vi "Drive Controller.vi"(8 "error in":errorcluster) -> ()   [LabVIEW 2015]
doc: "This VI executes continuously carrying out the current operation and responding to updates or new operation requests. It will often contain the timing or control code that is difficult to place directly in TeleOp. This VI generally opens all sensors and motors and isolates the rest of the robot code from knowing implementation details of how the operations are carried out."
uses:
  Drive Setpoints.ctl
  Drive Operations.ctl
  <vilib>/Rock Robotics/WPI/SafetyOutput/WPI_SafetyOutputConfigMenu.ctl
  <vilib>/Rock Robotics/WPI/RobotDrive/WPI_RobotDriveOpen2MotorWithTalon.vi
panel:
  in  "CMD Limit":dbl=0.07
  out "Setpoints":T1(graph)
  out "Current\nCmd":string
  # "Tip: It may be helpful to observe inputs and sensor values.\nYou may also want to display tuning or debugging controls."
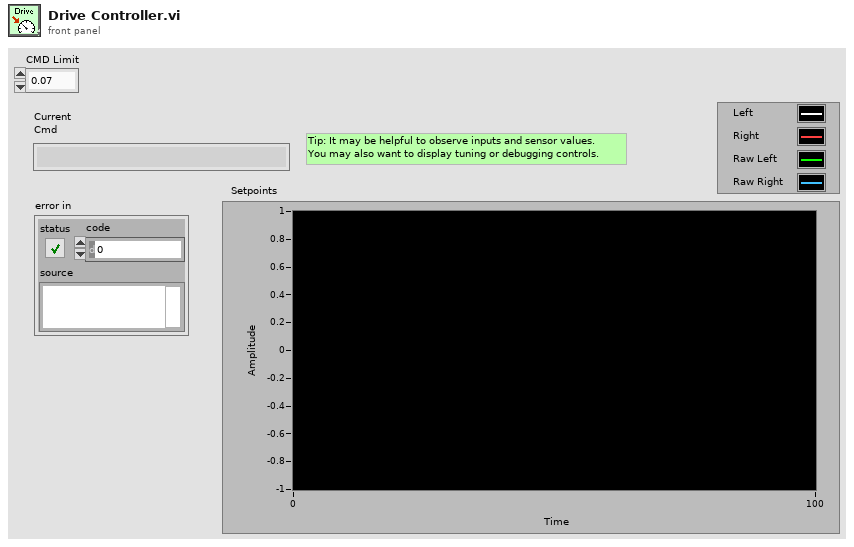
[diagram p1: front panel]
types:
  T1 = cluster{"Don't move motors while reserved":dbl, "Don't move motors while reserved":dbl, "Left Setpoint":dbl, "Right Setpoint":dbl}
  T2 = typedef "WPI_SafetyOutputConfigMenu.ctl" = enum16{"Enable", "Disable"}
  T3 = typedef "Drive Setpoints.ctl" = cluster{"Operation":T4, "Left Setpoint":dbl, "Right Setpoint":dbl, "Duration":dbl, "Throttle Setpoint":dbl}
  T4 = typedef "Drive Operations.ctl" = enum16{"Reserve", "Read Current", "Immediate", "Drive for Time", "Drive for Distance"}
  T5 = typedef "WPI_RobotDriveDevRef.ctl" = cluster{"DevStatus":errorcluster, "Motors[]":T6[], "Square Inputs":bool, "Max Output":dbl}
  T6 = typedef "WPI_MotorControlDeviceRef.ctl" = cluster{"DeviceStatus":errorcluster, "Type":T7, "PWM":cluster{"PWM Channel":T8, "DeadBand":T9}, "CAN":cluster{"Device Number":u8, "Control Mode":T10, "Semaphore":T11, "Max Vout":dbl, "TalonSRX Control Mode":T12}, "Invert":bool}
  T7 = typedef "WPI_MotorControlType.ctl" = enum16{"PWM", "CAN", "CANTalonSRX"}
  T8 = typedef "FPGA_DIOPWMChannel.ctl" = enum8{"PWM 0", "PWM 1", "PWM 2", "PWM 3", "PWM 4", "PWM 5", "PWM 6", "PWM 7", "PWM 8", "PWM 9", "PWM MXP 0", "PWM MXP 1", "PWM MXP 2", "PWM MXP 3", "PWM MXP 4", "PWM MXP 5", "PWM MXP 6", "PWM MXP 7", "PWM MXP 8", "PWM MXP 9", "Invalid"}
  T9 = typedef "WPI_PWMDeadband.ctl" = cluster{"Name":string, "maxPositivePwm":i32, "minPositivePwm":i32, "centerPwm":i32, "maxNegativePwm":i32, "minNegativePwm":i32, "angularRange":u16}
  T10 = typedef "WPI_CANJaguar_ControlMode.ctl" = enum8{"Percent VBus", "Current", "Speed", "Position", "Voltage"}
  T11 = typedef "Semaphore RefNum" = refnum<k1>
  T12 = typedef "WPI_CANTalonSRX_APIControlMode.ctl" = enum8{"Percent VBus", "Speed", "Position", "Slave", "Unchanged / Invalid", "Voltage Compensation", "Current", "Motion Profile"}
  T13 = typedef "Command Status Info.ctl" = cluster{"Name":string, "Status":T14, "notifier out":T15}
  T14 = typedef "Completion Status.ctl" = enum16{"Successful", "Aborted", "Incomplete"}
  T15 = typedef "Completion Notifier.ctl" = refnum<notifier>
  T16 = cluster{"SubSystem Data":T3, cluster{"Start Time (ms)":u32, "Iterations":i32}, cluster{"Command Info":T13, "Description":string, "SubSystem Data":T3, "notifier out":refnum<notifier>, "Subsystem Name":string}}
  T17 = cluster{"SubSystem Data":T3, cluster{"Start Time (ms)":u32, "Iterations":i32}, "Default Command Arguments":cluster{"Command Info":T13, "Description":string, "SubSystem Data":T3, "notifier out":refnum<notifier>, "Subsystem Name":string}}
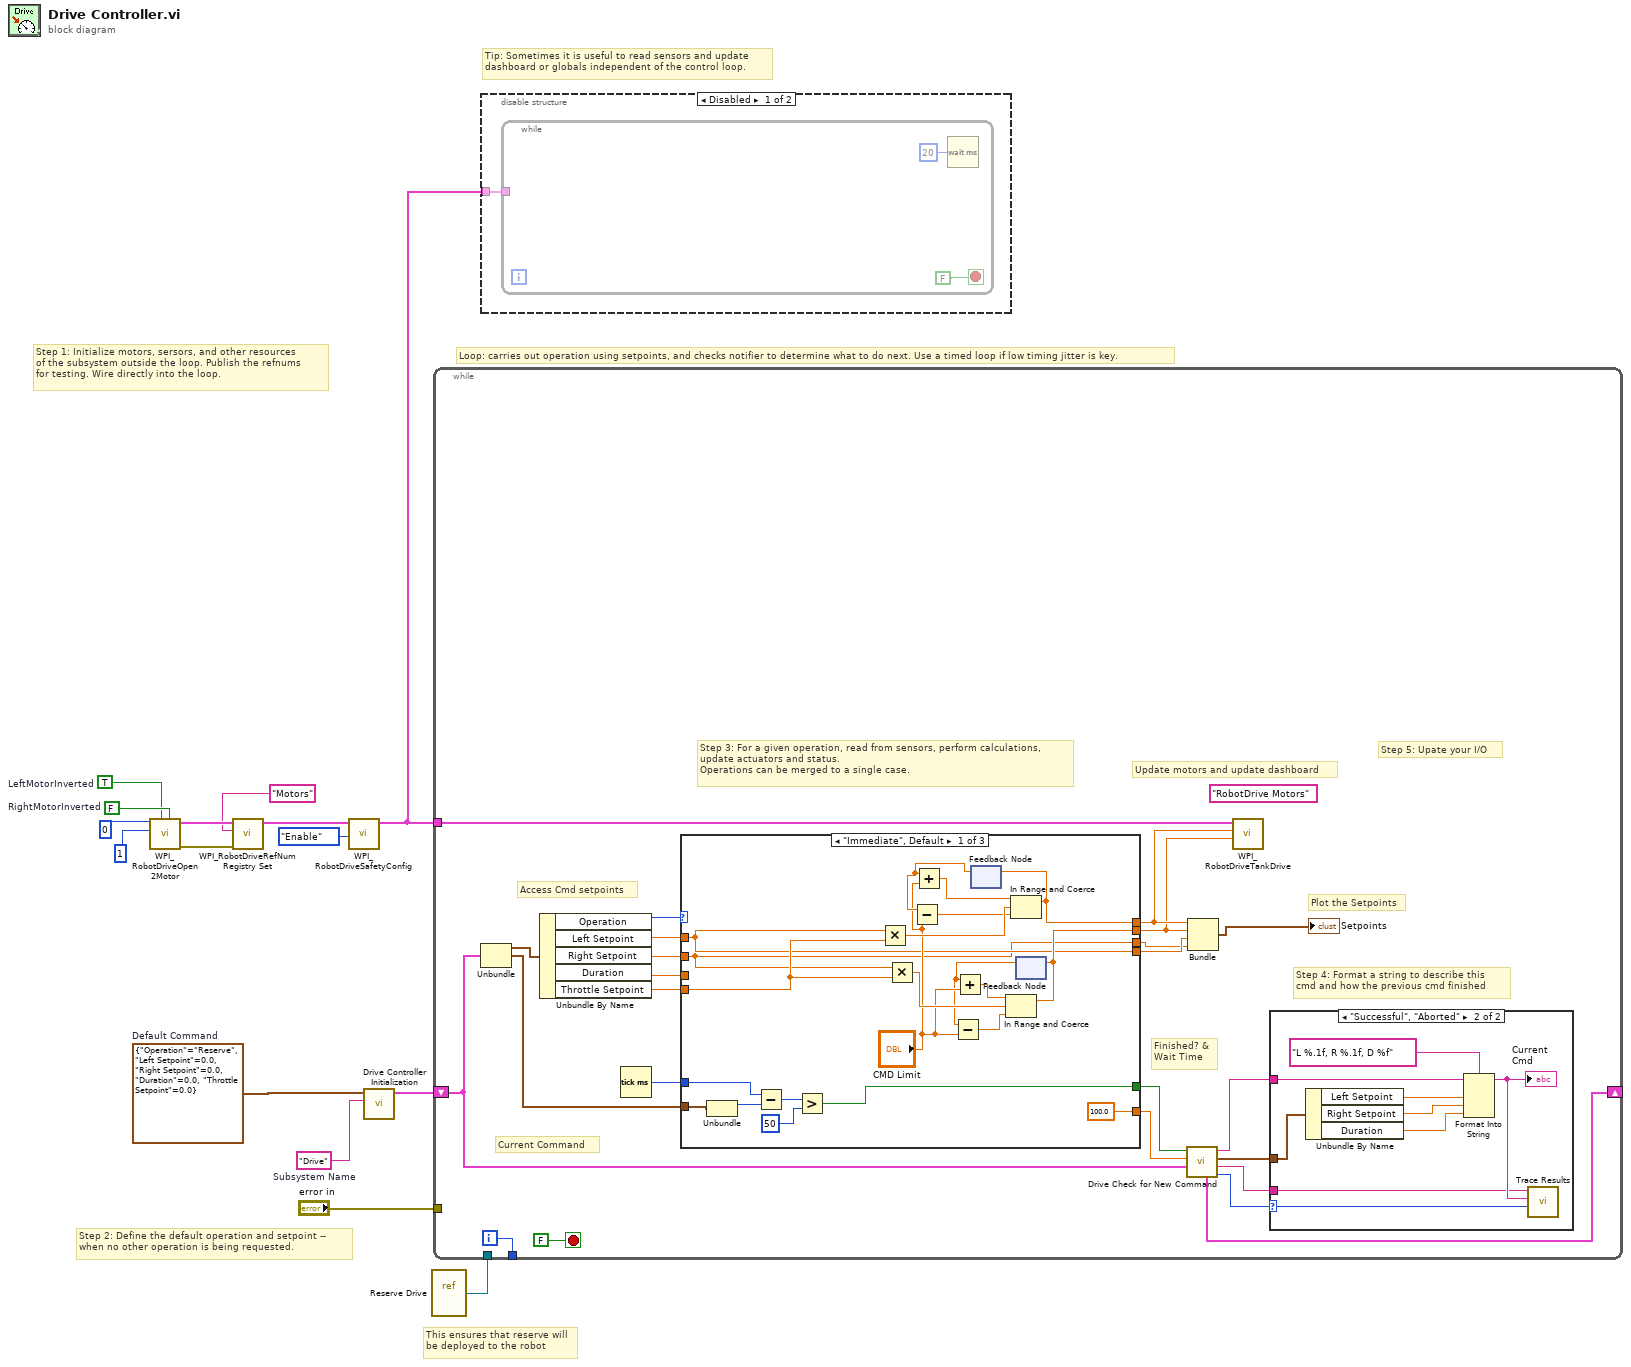
[diagram p0: block diagram]
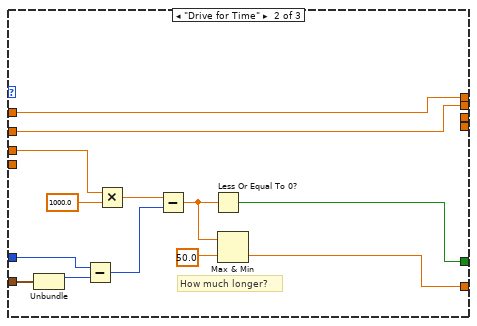
[diagram p4: hidden frame]
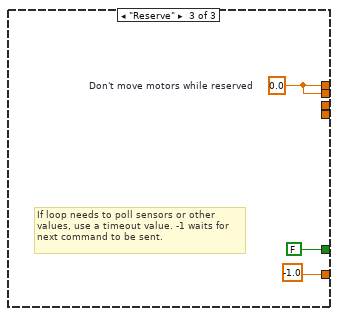
[diagram p5: hidden frame]
diagram:
  w10 = TRUE  # LeftMotorInverted
  w11 = FALSE  # RightMotorInverted
  w14 = T3 {"Operation"=enum."Reserve", "Left Setpoint"=0.0, "Right Setpoint"=0.0, "Duration"=0.0, "Throttle Setpoint"=0.0}  # Default Command
  w15 = "Drive"  # Subsystem Name
  # "This ensures that reserve will\nbe deployed to the robot"
  # "Tip: Sometimes it is useful to read sensors and update\ndashboard or globals independent of the control loop."
  # "Step 2: Define the default operation and setpoint --\nwhen no other operation is being requested."
  # "Step 1: Initialize motors, sersors, and other resources\nof the subsystem outside the loop. Publish the refnums\nfor testing. Wire directly into the loop."
  # "Loop: carries out operation using setpoints, and checks notifier to determine what to do next. Use a timed loop if low timing jitter is key."
  n1 = call-poly <vilib>:"WPI_RobotDriveOpen2Motor.vi"("Right Motor Inverted"=w11, "Left Motor Inverted"=w10, "Right Motor"=u8 1 ("Left Motor"), "Left Motor"=u8 0) -> ("error out"=w7:errorcluster, "RobotDriveDevRef"=w9:T5)  [unwired: 1 in, 5 out]
  n2 = call <vilib>:"WPI_RobotDriveRefNum Registry Set.vi"("error in (no error)"=w7, "refnum name"="Motors", "RobotDriveDevRef"=w9) -> ("RobotDriveDevRef"=w6:T5)  [unwired: 1 in, 7 out]
  n3 = call <vilib>:"WPI_RobotDriveSafetyConfig.vi"("mode"=WPI_SafetyOutputConfigMenu."Enable", "RobotDriveDevRef"=w6) -> ("RobotDriveDevRef"=w4:T5)  [unwired: 8 in, 1 out]
  n4 = call "Drive Controller Initialization.vi"("Subsystem Name"=w15, "Default Command"=w14) -> ("output cluster"=w2:T16)  [unwired: 9 in]
  n5 = vi-ref "Reserve Drive.vi"() -> (w1:refnum<vi>)
  n6 = while {
    shift-right: [w27] -> _
    shift-left: w2 -> [w20]
    tunnel: [w38] -> _
    tunnel: w4 -> [w35]
    tunnel: "error in" -> [_]
    tunnel: w1 -> [_]
    i -> [w38]
    stop <- FALSE stop-if-true
    (unwired) "RobotDrive Motors" ("Name")
    # "Step 5: Upate your I/O"
    # "Step 4: Format a string to describe this\ncmd and how the previous cmd finished"
    # "Current Command"
    # "Update motors and update dashboard"
    # "Plot the Setpoints"
    # "Access Cmd setpoints"
    # "Finished? &\nWait Time"
    # "Step 3: For a given operation, read from sensors, perform calculations,\nupdate actuators and status.\nOperations can be merged to a single case."
    n7 = Unbundle(w20) -> ("SubSystem Data"=w34:T3, w21:cluster{"Start Time (ms)":u32, "Iterations":i32})  [unwired: 1 out]
    n8 = Unbundle By Name(w34) -> ("Operation"=w33:T4, "Left Setpoint"=w32:dbl, "Right Setpoint"=w31:dbl, "Duration"=w30:dbl, "Throttle Setpoint"=w19:dbl)
    n9 = Tick Count (ms)() -> (millisecond timer value=w29:u32)
    n10 = case shown="\"Immediate\", Default" w33 {
      tunnel: [100.0 w70 -1.0] -> w26
      tunnel: [w64 w77 FALSE ("ignore previous (F)")] -> w25
      tunnel: w21 -> [w63 w79 _]
      tunnel: [w52 w76 w83] -> w37
      tunnel: [w51 w75 w83] -> w36
      tunnel: w32 -> [w50 w76 _]
      tunnel: w31 -> [w49 w75 _]
      tunnel: w30 -> [_ w74 _]
      tunnel: w29 -> [w65 w73 _]
      tunnel: w19 -> [w62 _ _]
      tunnel: [w50 _ _] -> w18
      tunnel: [w49 _ _] -> w17
      frame "Immediate", Default {
        n11 = Unbundle(w63) -> ("Start Time (ms)"=w66:u32)  [unwired: 1 out]
        n12 = Subtract(x=w65, y=w66) -> (x-y=w67:u32)
        n13 = Greater?(x=w67, y=u8 50 ("Left Motor")) -> (0:w64:bool)
        n14 = Multiply(x=w50, y=w62) -> (x*y=w61:dbl)
        n15 = Multiply(x=w49, y=w62) -> (x*y=w57:dbl)
        n16 = feedback #1() -> (w60:dbl)  [unwired: 1 in]
        n17 = Subtract(x=w60, y="CMD Limit") -> (x-y=w58:dbl)
        n18 = Add(x=w60, y="CMD Limit") -> (x+y=w59:dbl)
        n19 = In Range and Coerce(upper limit=w59, x=w61, lower limit=w58) -> (coerced(x)=w52:dbl)  [unwired: 1 out]
        n20 = feedback-in #1(w52) -> ()
        n21 = feedback #2() -> (w55:dbl)  [unwired: 1 in]
        n22 = Subtract(x=w55, y="CMD Limit") -> (x-y=w53:dbl)
        n23 = Add(x=w55, y="CMD Limit") -> (x+y=w54:dbl)
        n24 = In Range and Coerce(upper limit=w54, x=w57, lower limit=w53) -> (coerced(x)=w51:dbl)  [unwired: 1 out]
        n25 = feedback-in #2(w51) -> ()
      }
      frame "Drive for Time" {
        # "How much longer?"
        n26 = Unbundle(w79) -> ("Start Time (ms)"=w78:u32)  [unwired: 1 out]
        n27 = Subtract(x=w73, y=w78) -> (x-y=w82:u32)
        n28 = Multiply(x=w74, y=1000.0) -> (x*y=w81:dbl)
        n29 = Subtract(x=w81, y=w82) -> (x-y=w72:dbl)
        n30 = Less Or Equal To 0?(x=w72) -> (x <= 0?=w77:bool)
        n31 = Max & Min(x=w72, y=50.0) -> (min(x,y)=w70:dbl)  [unwired: 1 out]
      }
      frame "Reserve" {
        w83 = 0.0  # Don't move motors while reserved
        # "If loop needs to poll sensors or other\nvalues, use a timeout value. -1 waits for\nnext command to be sent."
      }
    }
    n32 = call "Drive Check for New Command.vi"("input cluster"=w20, "Wait time (ms)"=w26, "Finished?"=w25) -> ("Completion"=w28:T14, "Subsystem Name"=w22:string, "SetPoint"=w23:T3, "Initial Trace String"=w24:string, "output cluster"=w27:T17)  [unwired: 4 in]
    n33 = Bundle("Don't move motors while reserved"=w37, "Don't move motors while reserved"=w36, "Left Setpoint"=w18, "Right Setpoint"=w17) -> (→"Setpoints":T1)  [unwired: 1 in]
    n34 = call <vilib>:"WPI_RobotDriveTankDrive.vi"("Right axis value"=w36, "Left axis value"=w37, "RobotDriveDevRef"=w35) -> ()  [unwired: 6 in, 3 out]
    n35 = case shown="\"Successful\", \"Aborted\"" w28 {
      selector: w28 -> [_ w48]
      tunnel: w24 -> [_ w43]
      tunnel: w23 -> [_ w44]
      tunnel: w22 -> [_ w40]
      frame "Incomplete", Default {
        # "Continuing current command"
      }
      frame "Successful", "Aborted" {
        # "Report and setup for next command"
        n36 = Unbundle By Name(w44) -> ("Left Setpoint"=w46:dbl, "Right Setpoint"=w47:dbl, "Duration"=w41:dbl)
        n37 = Format Into String(format string="L %.1f, R %.1f, D %f", initial string=w43, w46, w47, w41) -> (resulting string=w42:string)  [unwired: 1 in, 1 out]
        "Current\nCmd" <- w42
        n38 = call <vilib>:"Trace Results.vi"("Status of previous command"=w48, "Description"=w42, "Subsystem"=w40) -> ()  [unwired: 9 in]
      }
    }
  }
  n39 = disable-structure shown="Disabled" {
    disable-tunnel: w4 -> [w86 _]
    frame Disabled {
      n40 = while {
        tunnel: w86 -> [_]
        stop <- FALSE stop-if-true
        n41 = Wait (ms)(milliseconds to wait=u32 20) -> ()  [unwired: 1 out]
      }
    }
    frame Enabled {
    }
  }
